vi "Read Factor time.vi"(11 "Collision in":refnum<class "Collision.lvclass">) -> (2 "Factor time":dbl)   [LabVIEW 2021, in "Collision.lvclass"]
doc: "MIT Licence\nCopyright (c) 2024 David Grollier"
uses:
  Collision.lvclass
  Collision.lvclass/Collision.ctl
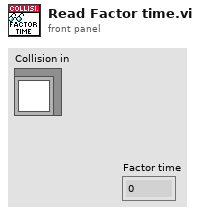
[diagram p1: front panel]
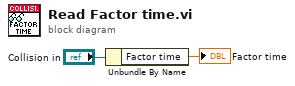
[diagram p0: block diagram]
diagram:
  n1 = Unbundle By Name("Collision in") -> ("Factor time"=→"Factor time":dbl)
